vi "getInfo.vi"(8 "error in (no error)":errorcluster, 11 "pHandle":u32) -> (0 "error out":errorcluster, 1 "firmwareVersion":string, 2 "pDeviceId":u32, 3 "productCode":string, 4 "calibDataVersion":string, 5 "mainBoardVersion":string, 6 "gpsBoardVersion":string, 7 "return type":i32)   [LabVIEW 2011, in "sbgLabView.lvlib"]
uses:
  sbgLabView.lvlib
  sbgMatLab.dll
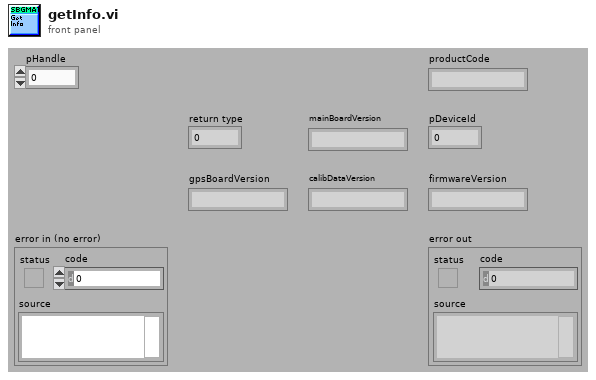
[diagram p1: front panel]
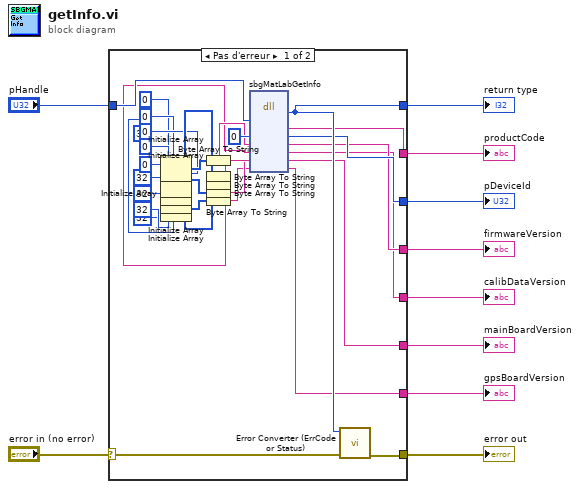
[diagram p0: block diagram]
diagram:
  n1 = case shown="Pas d'erreur" "error in (no error)" {
    selector: "error in (no error)" -> [w12 w42]
    tunnel: [w11 w42] -> w9
    tunnel: [w41 _] -> w8
    tunnel: "pHandle" -> [w40 _]
    tunnel: [w35 _] -> w6
    tunnel: [w33 _] -> w5
    tunnel: [w28 _] -> w4
    tunnel: [w23 _] -> w3
    tunnel: [w18 _] -> w2
    tunnel: [w13 _] -> w1
    frame No Error {
      n2 = Initialize Array(u8 0 ("element"), 32 ("dimension size")) -> (w39:u8[])
      n3 = Initialize Array(u8 0 ("element"), 32 ("dimension size")) -> (w32:u8[])
      n4 = Initialize Array(u8 0 ("element"), 32 ("dimension size")) -> (w27:u8[])
      n5 = Initialize Array(u8 0 ("element"), 32 ("dimension size")) -> (w22:u8[])
      n6 = Initialize Array(u8 0 ("element"), 32 ("dimension size")) -> (w17:u8[])
      n7 = Byte Array To String(unsigned byte array=w39) -> (string=w38:string)
      n8 = Byte Array To String(unsigned byte array=w32) -> (string=w31:string)
      n9 = Byte Array To String(unsigned byte array=w27) -> (string=w26:string)
      n10 = Byte Array To String(unsigned byte array=w22) -> (string=w21:string)
      n11 = Byte Array To String(unsigned byte array=w17) -> (string=w16:string)
      n12 = dll-call lib="C:/SBG-Systems/remote/projects/software/projects/labviewExample/sbgLabView/sbgMatLab.*" fn="sbgMatLabGetInfo"("pHandle"=w40, "productCode"=w38, "pDeviceId"=u32 0, "firmwareVersion"=w31, "calibDataVersion"=w26, "mainBoardVersion"=w21, "gpsBoardVersion"=w16) -> (w41:i32, "productCode"=w35:string, "pDeviceId"=w33:u32, "firmwareVersion"=w28:string, "calibDataVersion"=w23:string, "mainBoardVersion"=w18:string, "gpsBoardVersion"=w13:string)  [unwired: 4 in, 2 out]
      n13 = call "Error Converter (ErrCode or Status).vi"("error in (no error)"=w12, "error code"=w41) -> ("error out"=w11:errorcluster)  [unwired: 9 in]
    }
    frame Error {
    }
  }
  "return type" <- w8
  "productCode" <- w6
  "pDeviceId" <- w5
  "firmwareVersion" <- w4
  "calibDataVersion" <- w3
  "mainBoardVersion" <- w2
  "gpsBoardVersion" <- w1
  "error out" <- w9
